vi "XYIntGraph.vi"(1 "Columns":i32, 2 "Rows":i32, 3 "Z Intensity":dbl[](array[numeric]), 4 "XY Pos":dbl[][](array[numeric])) -> (0 "Intensity Graph":dbl[][](graph))   [LabVIEW 2019]
panel:
  in  "XY Pos 2":dbl[][](array[numeric])
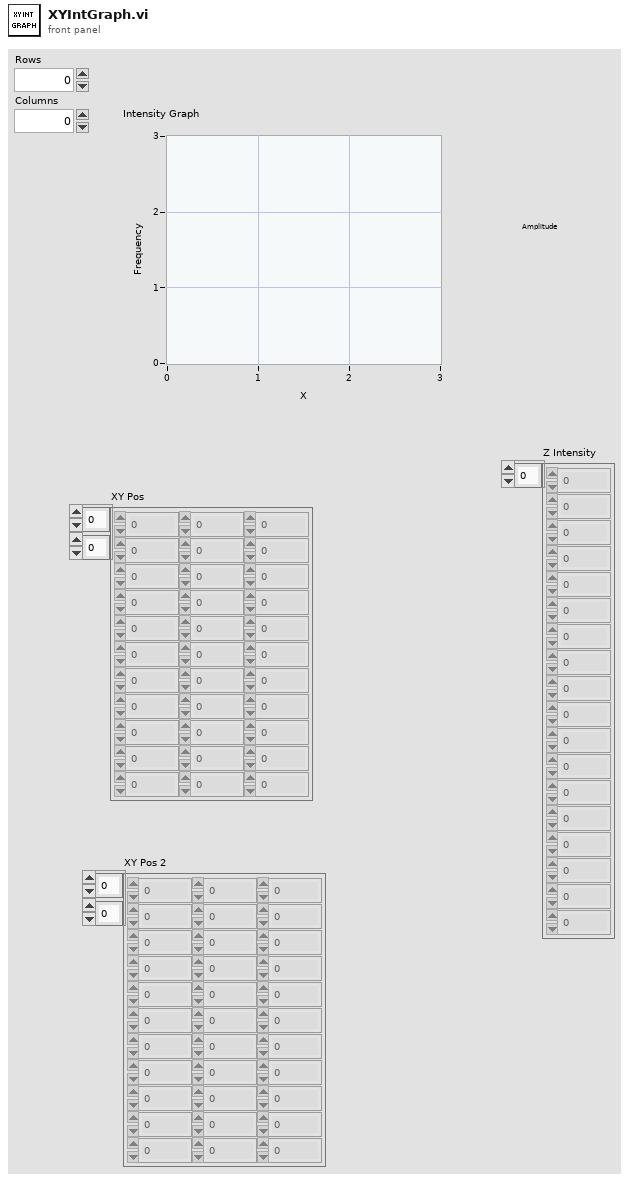
[diagram p1: front panel]
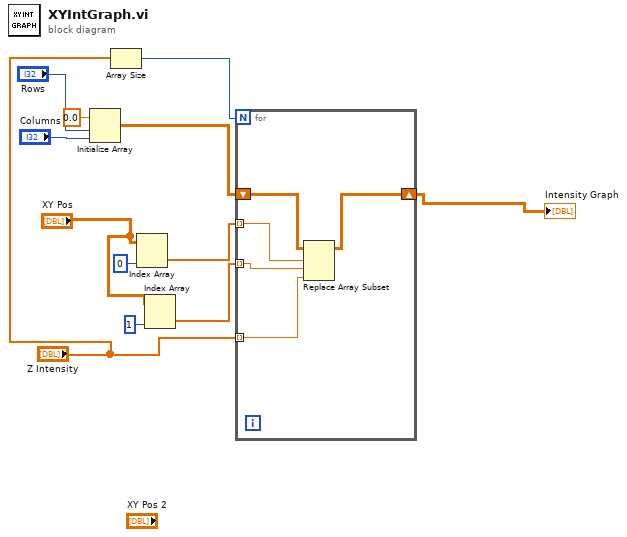
[diagram p0: block diagram]
diagram:
  n1 = Initialize Array(0.0 ("element"), "Rows", "Columns") -> (w9:dbl[][])
  n2 = Array Size(array="Z Intensity") -> (size(s)=w1:i32)
  n3 = Index Array(array="XY Pos", index (col)=0 ("disabled index (col)")) -> (element=w5:dbl[])  [unwired: 1 in]
  n4 = Index Array(array="XY Pos", index (col)=1 ("disabled index (col)")) -> (element=w4:dbl[])  [unwired: 1 in]
  n5 = for {
    N: w1 -> [_]
    shift-right: [w16] -> w3
    shift-left: w9 -> [w17]
    tunnel: w5 -> [w15] mode=indexing
    tunnel: w4 -> [w14] mode=indexing
    tunnel: "Z Intensity" -> [w13] mode=indexing
    n6 = Replace Array Subset(array=w17, new element=w13, index (row)=w15, index (col)=w14) -> (w16:dbl[][])
  }
  "Intensity Graph" <- w3
